vi "DestroyProtectedEvents.vi"(8 "error in (no error)":errorcluster, 11 "SMO.UI.Splash":refnum<class "SMO.UI.Splash.lvclass">) -> (0 "error out":errorcluster, 3 "SMO.UI.Splash out":refnum<class "SMO.UI.Splash.lvclass">)   [LabVIEW 2013, in "SMO.UI.Splash.lvclass"]
doc: "JKI State Machine Objects (SMO) 1.0.0.5\nJKI - JKI\nCopyright (c) 2016, JKI"
uses:
  SMO.UI.Splash.lvclass
  <vilib>/JKI/JKI SMO/SMO.UI/SMO.UI.lvclass
panel:
  # "For instructions on how to use the JKI State Machine Objects, examples and video tutorials, visit:\nhttp://jki.net/state-machine-objects/\n\nJKI State Machine Objects™\nhttp://jki.net/state-machine-objects/\nCopyright (C) 2005-2015, JKI <info@jki.net>\nALL RIGHTS RESERVED"
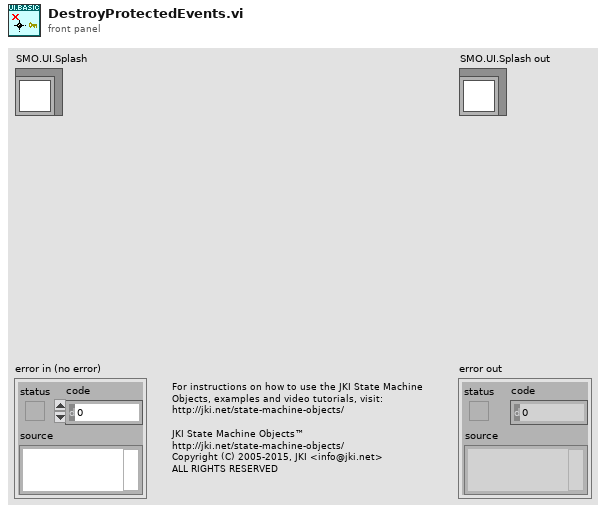
[diagram p1: front panel]
types:
  T1 = typedef "SMO.UI.Splash.lvclass/ProtectedEvents--Cluster.ctl" = cluster{"Display Message":T2}
  T2 = typedef "SMO.UI.Splash.lvclass/DisplayMessage--Cluster.ctl" = refnum<user-event>
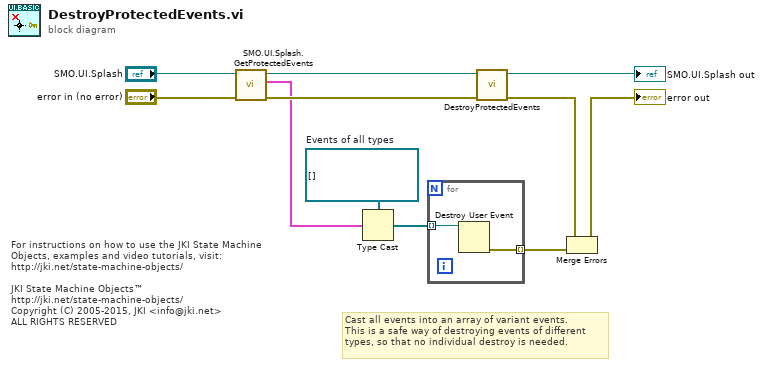
[diagram p0: block diagram]
diagram:
  w9 = refnum<user-event>[] []  # Events of all types
  # "For instructions on how to use the JKI State Machine Objects, examples and video tutorials, visit:\nhttp://jki.net/state-machine-objects/\n\nJKI State Machine Objects™\nhttp://jki.net/state-machine-objects/\nCopyright (C) 2005-2015, JKI <info@jki.net>\nALL RIGHTS RESERVED"
  # "Cast all events into an array of variant events.\nThis is a safe way of destroying events of different\ntypes, so that no individual destroy is needed."
  n1 = call "SMO.UI.Splash.GetProtectedEvents.vi"("error in (no error)"="error in (no error)", "SMO.UI.Splash in"="SMO.UI.Splash") -> ("error out"=w3:errorcluster, "Protected Events"=w2:T1, "SMO.UI.Splash out"=w5:refnum<class "SMO.UI.Splash.lvclass">)  [unwired: 7 in]
  n2 = Type Cast(type=w9, x=w2) -> (*(type *) &x=w10:refnum<user-event>[])
  n3 = for {
    tunnel: w10 -> [w13] mode=indexing
    tunnel: [w12] -> w11 mode=indexing
    n4 = Destroy User Event(user event=w13) -> (error out=w12:errorcluster)  [unwired: 1 in]
  }
  n5 = call-parent "DestroyProtectedEvents.vi"("error in (no error)"=w3, "SMO"=w5) -> ("error out"=w8:errorcluster, "SMO out"=→"SMO.UI.Splash out":refnum<class "SMO.UI.Splash.lvclass">)  [unwired: 8 in]
  n6 = Merge Errors(w8, w11) -> (→"error out":errorcluster)
